vi "Exit.vi"(7 "Shared Library":path=path "C:/Program Files/libssh2/bin/libssh2.dll", 8 "Error In":errorcluster) -> (0 "Error Out":errorcluster)   [LabVIEW 2017, in "LabSSH2.lvlib"]
uses:
  LabSSH2.lvlib
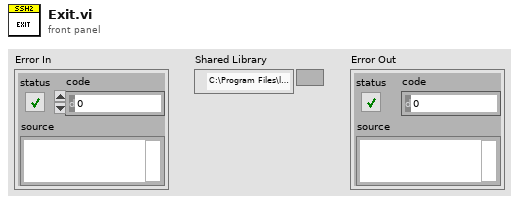
[diagram p1: front panel]
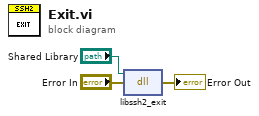
[diagram p0: block diagram]
diagram:
  n1 = dll-call lib="C:/Program Files/libssh2/bin/libssh2.dll" fn="libssh2_exit"(path in="Shared Library", error in="Error In") -> (error out=→"Error Out":errorcluster)  [unwired: 2 in, 1 out]
